vi "ScaleSensor.vi"(11 "value":i32) -> (3 "scaled value":u16)   [LabVIEW 2019]
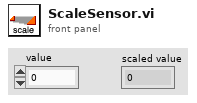
[diagram p1: front panel]
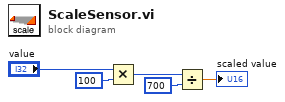
[diagram p0: block diagram]
diagram:
  n1 = Multiply(x="value", y=100 ("value")) -> (x*y=w2:i32)
  n2 = Divide(x=w2, y=700 ("value")) -> (x/y=→"scaled value":dbl)
